vi "Read From CSV w Presentation Column.vi"(8 "Error In":errorcluster, 11 "Spreadsheet path (.csv)":path=path "C:/Users/husmith/Desktop/MyData.csv") -> (0 "Error Out":errorcluster, 1 "Gestation":string, 2 "Presentation Values":string[](array[string]), 3 "Data":dbl[][](array[numeric]))   [LabVIEW 2017]
uses:
  <vilib>/Utility/file.llb/Read Delimited Spreadsheet (string).vi
  <vilib>/Utility/file.llb/Read Delimited Spreadsheet (DBL).vi
panel:
  out "Number of columns":i32
  out "String Display":string[][](array[string])
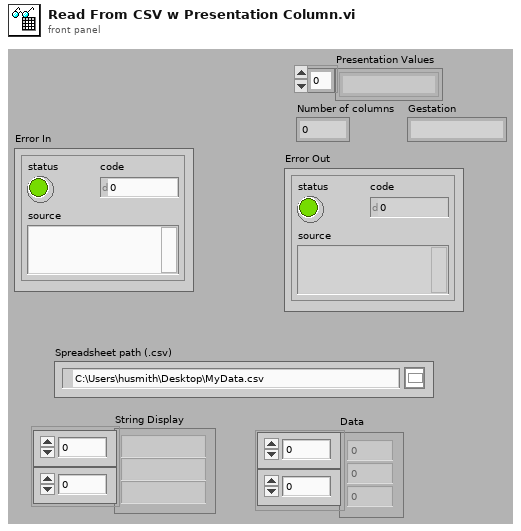
[diagram p1: front panel]
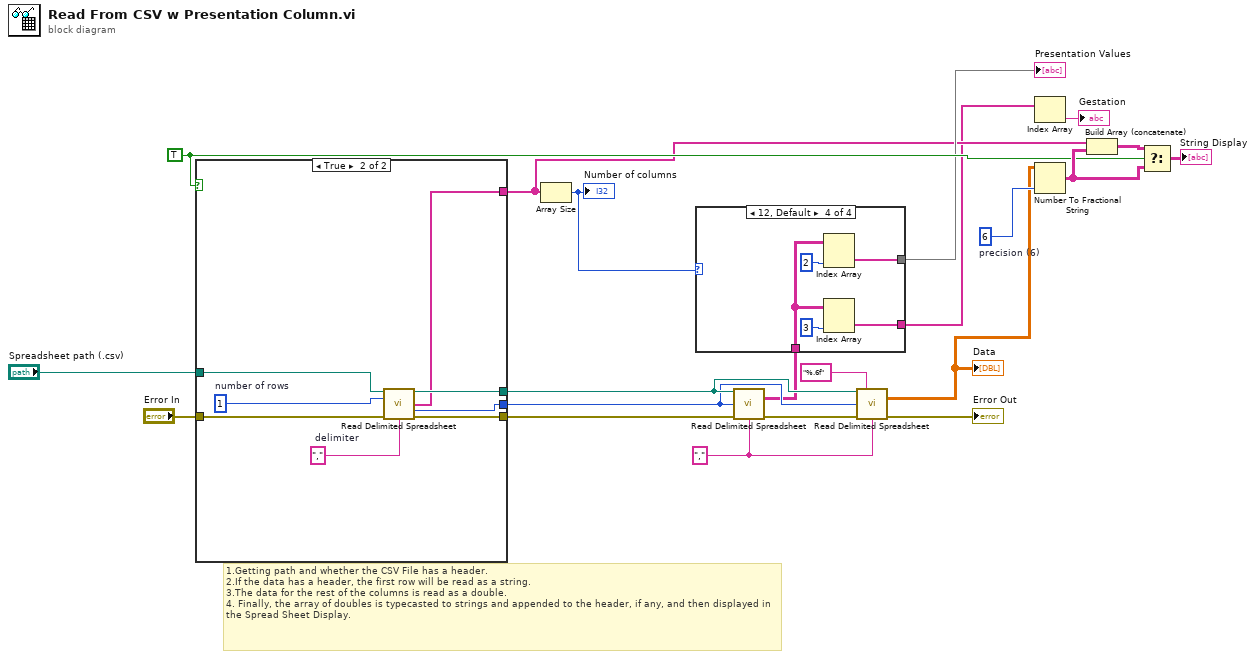
[diagram p0: block diagram]
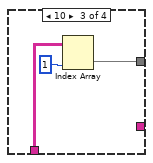
[diagram p4: hidden frame]
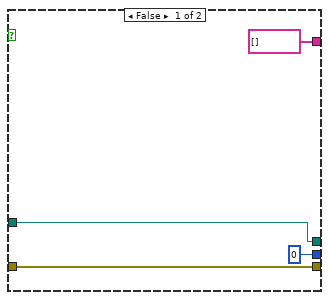
[diagram p5: hidden frame]
diagram:
  w3 = "," ("delimiter (\\t)")
  w13 = TRUE ("Headers?")
  w17 = i16 6  # precision (6)
  # "1.Getting path and whether the CSV File has a header.\n2.If the data has a header, the first row will be read as a string.\n3.The data for the rest of the columns is read as a double.\n4. Finally, the array of doubles is typecasted to strings and appended to the header, if any, and then displayed in the Spread Sheet Display."
  n1 = case shown="True" w13 {
    tunnel: "Spreadsheet path (.csv)" -> [w23 w33]
    tunnel: [string[] [] ("first row") w29] -> w8
    tunnel: [0 ("mark after read (chars.)") w28] -> w14
    tunnel: [w23 w32] -> w16
    tunnel: [w22 w27] -> w10
    tunnel: "Error In" -> [w22 w26]
    frame False {
    }
    frame True {
      w31 = 1  # number of rows
      w30 = ","  # delimiter
      n2 = call-poly <vilib>:"Read Delimited Spreadsheet.vi"("file path (dialog if empty)"=w33, "number of rows (all:-1)"=w31, "error in (no error)"=w26, "delimiter (\\t)"=w30) -> ("new file path (Not A Path if cancelled)"=w32:path, "first row"=w29:string[], "mark after read (chars.)"=w28:i32, "error out"=w27:errorcluster)  [unwired: 6 in, 2 out]
    }
  }
  n3 = Array Size(array=w8) -> (size(s)=w1:i32)
  "Number of columns" <- w1
  n4 = call-poly <vilib>:"Read Delimited Spreadsheet.vi"("file path (dialog if empty)"=w16, "start of read offset (chars.:0)"=w14, "error in (no error)"=w10, "delimiter (\\t)"=w3) -> ("all rows"=w2:string[][], "error out"=w4:errorcluster)  [unwired: 6 in, 4 out]
  n5 = case shown="12, Default" w1 {
    tunnel: [_ _ w36 w41] -> w9
    tunnel: [_ _ _ w40] -> w7
    tunnel: w2 -> [_ _ w34 w38]
    frame 7 {
      # "frame, x, y, z, pitch, yaw, roll"
    }
    frame 9 {
      # "frame, x, y, z, qx, qy, qz, qw, tracked?"
    }
    frame 10 {
      n6 = Index Array(array=w34, index (col)=1 ("disabled index (col)")) -> (element=w36:string[])  [unwired: 1 in]
    }
    frame 12, Default {
      n7 = Index Array(array=w38, index (col)=2 ("disabled index (col)")) -> (element=w41:string[])  [unwired: 1 in]
      n8 = Index Array(array=w38, index (col)=3 ("disabled index (col)")) -> (element=w40:string[])  [unwired: 1 in]
    }
  }
  "Presentation Values" <- w9
  n9 = call-poly <vilib>:"Read Delimited Spreadsheet.vi"("file path (dialog if empty)"=w16, "format (%.3f)"="%.6f", "start of read offset (chars.:0)"=w14, "error in (no error)"=w4, "delimiter (\\t)"=w3) -> ("all rows"=w15:dbl[][], "error out"=→"Error Out":errorcluster)  [unwired: 5 in, 4 out]
  "Data" <- w15
  n10 = Index Array(array=w7) -> (element=→"Gestation":string)  [unwired: 1 in]
  n11 = Number To Fractional String(number=w15, precision (6)=w17) -> (F-format string=w18:string[][])  [unwired: 2 in]
  n12 = Build Array (concatenate)(w8, w18) -> (w20:string[][])
  n13 = Select(t=w20, s=w13, f=w18) -> (s? t:f=→"String Display":string[][])
